vi "ROI entry screen-Replicate ROI.vi"(8 "error in (no error)":errorcluster, 10 "New Z plane":i32, 11 "XYZ":T3 {"Apparent Frame Size" format="%#_6f"; "Original FOV (um)" format="%#_6f"; "Pixels per miniscan" format="%#_6f"; "Dwell Time per pixel" format="%#_6f"; "Resolution" format="%#_6f"; "ROI group ID" format="%#_6f"; "Laser Power (%)" format="%#_6f"; "Zoom" format="%#_6f"; "Frame Size" format="%#_6f"; "Number of lines" format="%#_6f"; "Composite ID" format="%#_6f"; "Angle (deg)" format="%#_6f"; "ROI Time (ns)" format="%#_6f"; "ROI ID" format="%#_6f"; "Pixels in ROI" format="%#_6f"; "ROI index" format="%#_6f"; "Z stop" format="%#_6f"; "Y stop" format="%#_6f"; "X stop" format="%#_6f"; "Z start" format="%#_6f"; "X start" format="%#_6f"; "Y start" format="%#_6f"}) -> (0 "error out":errorcluster, 3 "ROI info":T1={"ROI Enum"=enum."Point", "Coordinates"=[], "Zoom"=1.0, "POI Dwell time"=1.0, "Rel. Resolution"=1.0, "Laser Power"=1.0, "Frame Size"=1.0, "FOV"=1.0, "Z start"=0.0, "Z stop"=0.0, "Z planeIdx(s)"=[], "Z planecodes(s)"=[]} {"FOV" min=1.0 max=10.0 step=1.0; "Frame Size" min=1.0 max=10.0 step=1.0; "Laser Power" min=1.0 max=10.0 step=0.10000000149011612; "Rel. Resolution" min=1.0 max=10.0 step=1.0; "POI Dwell time" min=1.0 max=10.0 step=0.10000000149011612; "Zoom" min=1.0 max=10.0 step=0.10000000149011612})   [LabVIEW 2020]
uses:
  Visualisation/Functional Imaging Viewer/Typedefs/ROI parameters data type.ctl
  Typedefs/ROI spec.ctl
  Typedefs/ROI ID Enum.ctl
  Typedefs/Redraw ROI.ctl
  Typedefs/ROI management FG states.ctl
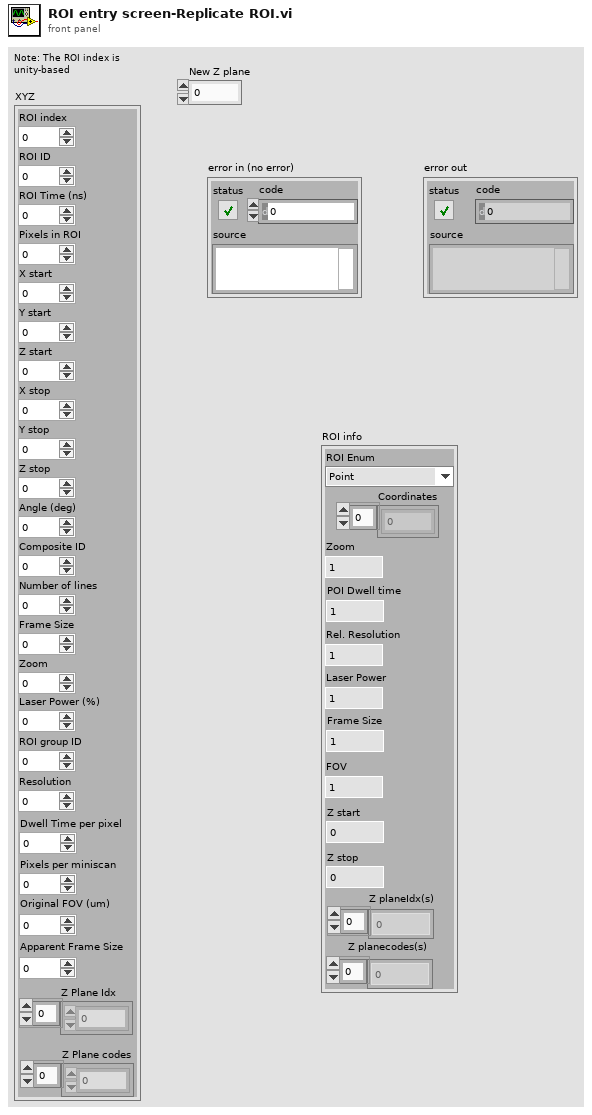
[diagram p1: front panel]
types:
  T1 = typedef "ROI spec.ctl" = cluster{"ROI Enum":T2, "Coordinates":i32[], "Zoom":dbl, "POI Dwell time":dbl, "Rel. Resolution":dbl, "Laser Power":dbl, "Frame Size":dbl, "FOV":dbl, "Z start":dbl, "Z stop":dbl, "Z planeIdx(s)":i32[], "Z planecodes(s)":u8[]}
  T2 = typedef "ROI ID Enum.ctl" = enum16{"Point", "MiniScan", "Comp. MiniScan", "Rectangle", "Comp. volume", "Arb. plane point", "None"}
  T3 = typedef "ROI parameters data type.ctl" = cluster{"ROI index":dbl, "ROI ID":dbl, "ROI Time (ns)":dbl, "Pixels in ROI":dbl, "X start":dbl, "Y start":dbl, "Z start":dbl, "X stop":dbl, "Y stop":dbl, "Z stop":dbl, "Angle (deg)":dbl, "Composite ID":dbl, "Number of lines":dbl, "Frame Size":dbl, "Zoom":dbl, "Laser Power (%)":dbl, "ROI group ID":dbl, "Resolution":dbl, "Dwell Time per pixel":dbl, "Pixels per miniscan":dbl, "Original FOV (um)":dbl, "Apparent Frame Size":dbl, "Z Plane Idx":i32[], "Z Plane codes":i32[]}
  T4 = typedef "ROI management FG states.ctl" = enum16{"Read", "Write", "Write-from dataset", "Clear Last", "Clear All", "Delete ROI", "Update ROIs time", "Reload last ROI set", "Modify ROI Parameters", "Offset all ROI", "Offset visible ROI", "Modify Dwell Time", "Modify Laser Power"}
  T5 = typedef "Redraw ROI.ctl" = enum16{"Redraw All", "Redraw Deselected", "Draw Last", "Redraw Selected"}
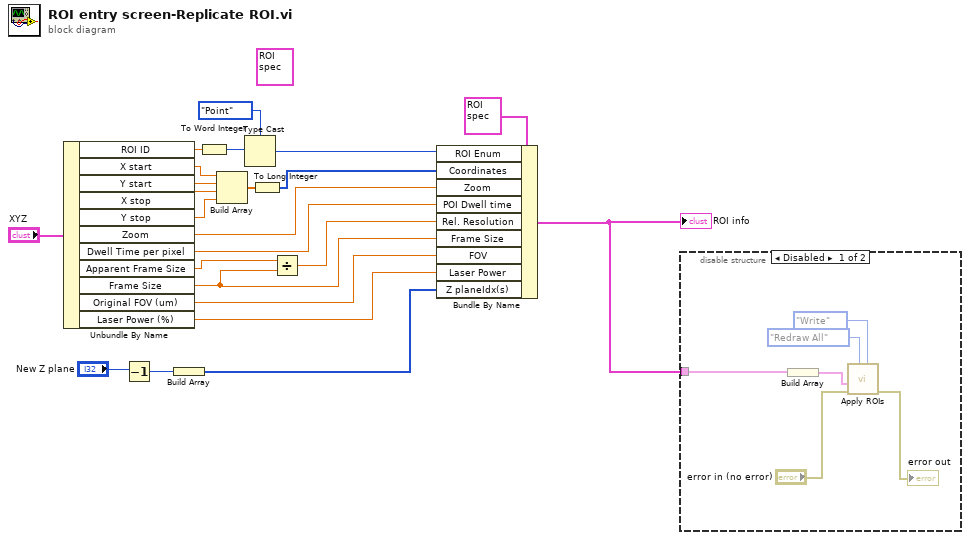
[diagram p0: block diagram]
diagram:
  (unwired) T1 {"ROI Enum"=enum."Point", "Coordinates"=[], "Zoom"=1.0, "POI Dwell time"=1.0, "Rel. Resolution"=1.0, "Laser Power"=1.0, "Frame Size"=1.0, "FOV"=1.0, "Z start"=0.0, "Z stop"=0.0, "Z planeIdx(s)"=[], "Z planecodes(s)"=[]} ("ROI Info")
  n1 = Unbundle By Name("XYZ") -> ("ROI ID"=w22:dbl, "X start"=w18:dbl, "Y start"=w17:dbl, "X stop"=w16:dbl, "Y stop"=w15:dbl, "Zoom"=w12:dbl, "Dwell Time per pixel"=w11:dbl, "Apparent Frame Size"=w5:dbl, "Frame Size"=w3:dbl, "Original FOV (um)"=w2:dbl, "Laser Power (%)"=w1:dbl)
  n2 = Decrement(x="New Z plane") -> (x-1=w8:i32)
  n3 = Build Array(w8) -> (w10:i32[])
  n4 = To Word Integer(number=w22) -> (16bit integer=w21:i16)
  n5 = Build Array(w18, w17, w16, w15) -> (w14:dbl[])
  n6 = Type Cast(type=ROI_ID_Enum."Point" ("ROI Enum"), x=w21) -> (*(type *) &x=w19:T2)
  n7 = To Long Integer(number=w14) -> (32bit integer=w13:i32[])
  n8 = Divide(x=w5, y=w3) -> (x/y=w4:dbl)
  n9 = Bundle By Name(cluster=T1 {"ROI Enum"=enum."Point", "Coordinates"=[], "Zoom"=0.0, "POI Dwell time"=1.0, "Rel. Resolution"=1.0, "Laser Power"=1.0, "Frame Size"=1.0, "FOV"=1.0, "Z start"=0.0, "Z stop"=0.0, "Z planeIdx(s)"=[], "Z planecodes(s)"=[]}, "ROI Enum"=w19, "Coordinates"=w13, "Zoom"=w12, "POI Dwell time"=w11, "Rel. Resolution"=w4, "Frame Size"=w3, "FOV"=w2, "Laser Power"=w1, "Z planeIdx(s)"=w10) -> (w9:T1)
  "ROI info" <- w9
  n10 = disable-structure shown="Disabled" {
    disable-tunnel: w9 -> [w29 _]
    frame Disabled {
      n11 = Build Array(w29) -> (w28:T1[])
      n12 = call "Apply ROIs.vi"("Function"=ROI_management_FG_states."Write", "Mode (Redraw All)"=Redraw_ROI."Redraw All", "error in (no error)"="error in (no error)", "ROIs Info []"=w28) -> ("error out"=→"error out":errorcluster)  [unwired: 5 in, 2 out]
    }
    frame Enabled {
    }
  }
